vi "Send Image Data.vi"(0 "Connection In":refnum<k5>, 7 "Image Data":T1, 11 "Error In":errorcluster) -> (4 "Connection Out":refnum<k5>, 8 "Success":bool, 15 "Error Out":errorcluster)   [LabVIEW 2016]
uses:
  Orca Flash Data Spooler/Orca Data Spooler Type Defs/Orca Data Spooler Transfer Data.ctl
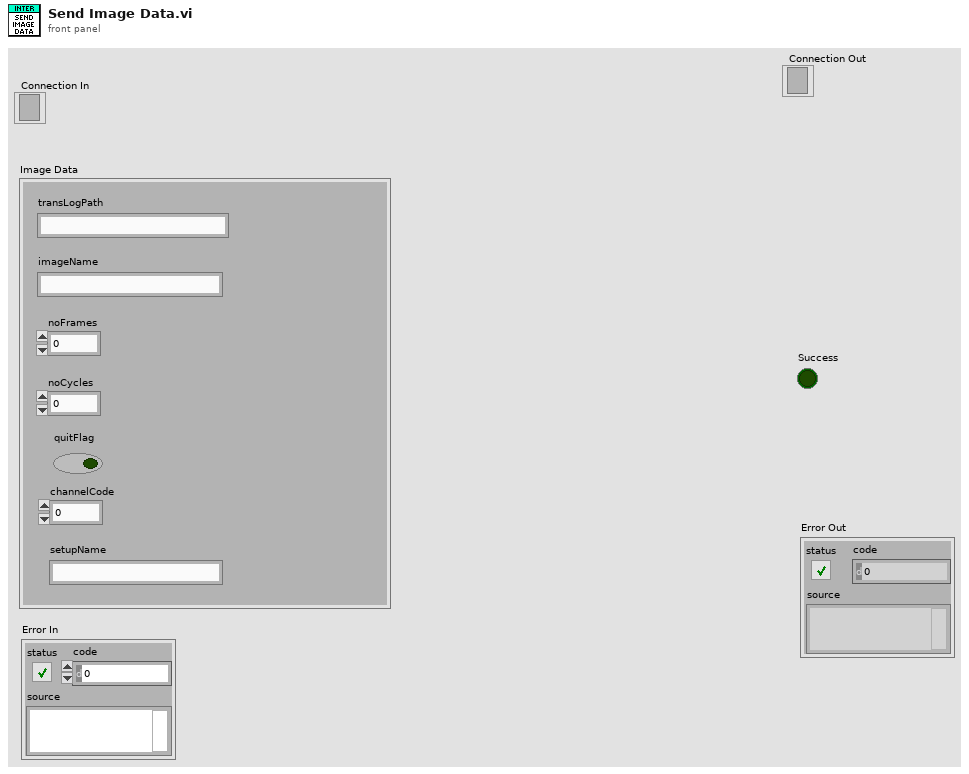
[diagram p1: front panel]
types:
  T1 = typedef "Orca Data Spooler Transfer Data.ctl" = cluster{"transLogPath":string, "imageName":string, "noFrames":u32, "noCycles":u16, "quitFlag":bool, "channelCode":u8, "setupName":string}
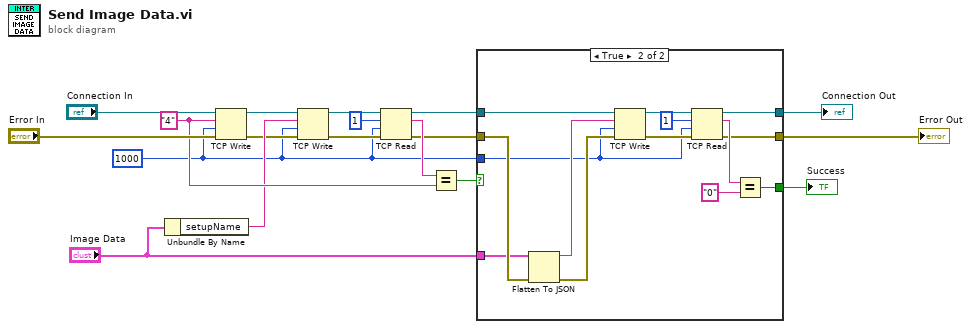
[diagram p0: block diagram]
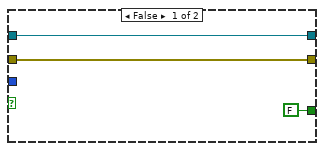
[diagram p2: hidden frame]
diagram:
  w14 = "4" ("data in")
  w1 = 1000 ("timeout ms (25000)")
  n1 = Unbundle By Name("Image Data") -> ("setupName"=w5:string)
  n2 = TCP Write(connection ID="Connection In", data in=w14, error in (no error)="Error In", 9:w1) -> (connection ID out=w6:refnum<k5>, error out=w4:errorcluster)  [unwired: 1 out]
  n3 = TCP Write(connection ID=w6, data in=w5, error in (no error)=w4, 9:w1) -> (connection ID out=w3:refnum<k5>, error out=w2:errorcluster)  [unwired: 1 out]
  n4 = TCP Read(connection ID=w3, bytes to read=1, error in (no error)=w2, 9:w1) -> (connection ID out=w12:refnum<k5>, data out=w15:string, error out=w11:errorcluster)  [unwired: 1 in]
  n5 = Equal?(x=w15, y=w14) -> (x = y?=w13:bool)
  n6 = case shown="True" w13 {
    tunnel: w12 -> [w21 w35]
    tunnel: w11 -> [w20 w34]
    tunnel: w1 -> [_ w28]
    tunnel: [w20 w25] -> w9
    tunnel: [w21 w24] -> w10
    tunnel: [FALSE w23] -> w8
    tunnel: "Image Data" -> [_ w22]
    frame False {
    }
    frame True {
      n7 = Flatten To JSON(anything=w22, error in (no error)=w34) -> (JSON string=w32:string, 11:w33:errorcluster)  [unwired: 1 in]
      n8 = TCP Write(connection ID=w35, data in=w32, error in (no error)=w33, 9:w28) -> (connection ID out=w30:refnum<k5>, error out=w29:errorcluster)  [unwired: 1 out]
      n9 = TCP Read(connection ID=w30, bytes to read=1, error in (no error)=w29, 9:w28) -> (connection ID out=w24:refnum<k5>, data out=w27:string, error out=w25:errorcluster)  [unwired: 1 in]
      n10 = Equal?(x=w27, y="0") -> (x = y?=w23:bool)
    }
  }
  "Error Out" <- w9
  "Connection Out" <- w10
  "Success" <- w8
